vi "LWXPS_PositionerCompensationPreFeedForwardFrequencyNotchFilterGet.vi"(0 "XPS Reference IN":refnum<k24>, 5 "Positioner Name":string, 9 "Notch Frequency Number":i32, 11 "LabVIEW error IN":errorcluster) -> (3 "XPS Reference OUT":refnum<k24>, 4 "Returned error code":i32, 6 "Notch Frequency":dbl, 8 "Notch Bandwidth":dbl, 10 "Notch Gain":dbl, 14 "LabVIEW error OUT":errorcluster, 15 "XPS Error String":string)   [LabVIEW 2014]
uses:
  D:/XPSQ8_LabView_Library/Development/Source/Dll/Newport.XPS.CommandInterface.dll
  Dll/Newport.XPS.CommandInterface.dll
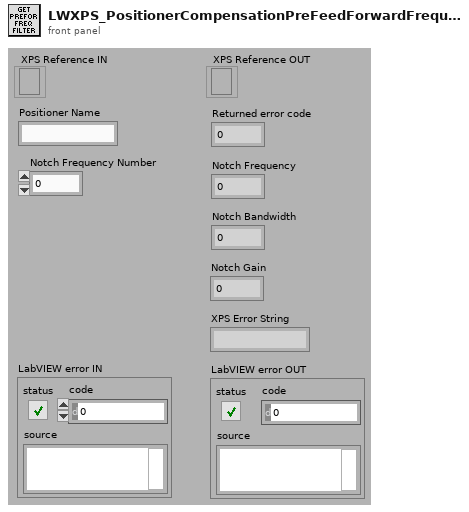
[diagram p1: front panel]
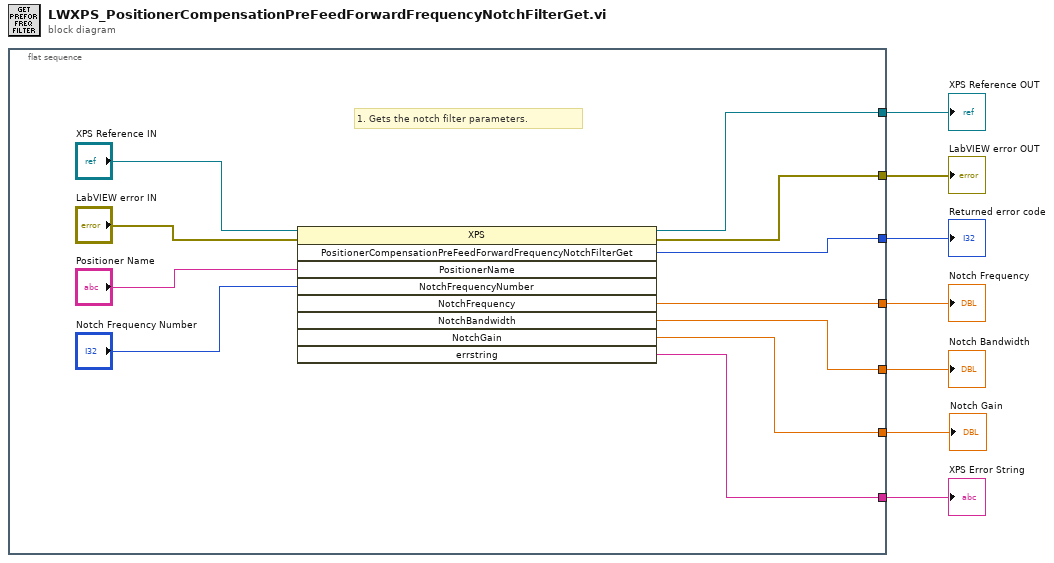
[diagram p0: block diagram]
diagram:
  n1 = flat-sequence {
    tunnel: [w16] -> w7
    tunnel: [w10] -> w6
    tunnel: [w17] -> w5
    tunnel: [w13] -> w4
    tunnel: [w12] -> w3
    tunnel: [w8] -> w2
    tunnel: [w11] -> w1
    frame #0 {
      # "1. Gets the notch filter parameters."
      n2 = invoke class="XPS" method="PositionerCompensationPreFeedForwardFrequencyNotchFilterGet"(reference="XPS Reference IN", error in="LabVIEW error IN", "PositionerName"="Positioner Name", "NotchFrequencyNumber"="Notch Frequency Number") -> (reference out=w16:refnum<k24>, error out=w10:errorcluster, "PositionerCompensationPreFeedForwardFrequencyNotchFilterGet"=w17:i32, "NotchFrequency"=w13:dbl, "NotchBandwidth"=w12:dbl, "NotchGain"=w11:dbl, "errstring"=w8:string)  [unwired: 5 in, 2 out]
    }
  }
  "XPS Error String" <- w2
  "XPS Reference OUT" <- w7
  "LabVIEW error OUT" <- w6
  "Returned error code" <- w5
  "Notch Frequency" <- w4
  "Notch Bandwidth" <- w3
  "Notch Gain" <- w1
